vi "sid_output.vi"(6 "inputValid":bool, 7 "startId":bool, 9 "sysIdParams":T1={"sysIdOutputRate"=100, "sysIdWaveSize"=4092, "sysIdRepetitions"=50} {"sysIdOutputRate" min=10}, 11 "feedbackHeight":fxp<+/-,28,1>) -> (0 "sysIdRunning":bool, 1 "recordPoint":bool, 2 "sysIdRep":u16, 3 "sid.o.height":fxp<+/-,28,1>, 4 "outputValid":bool)   [LabVIEW 2016]
uses:
  <vilib>/rvi/DataTransferAndStorage/Container/XNode/niFpgaContainer.xnode
  <instrlib>/_niInstr/Basic Elements/v1/FPGA/niInstr Basic Elements v1 FPGA.lvlib
  <vilib>/rvi/FXPMathLib/FxpAdd/XNode/nifxpmath_Add.xnode
  <vilib>/rvi/FXPMathLib/sim/FxpSim.dll
  <vilib>/rvi/FXPMathLib/FxpInterpret/XNode/nifxpmath_Interpret.xnode
  <vilib>/rvi/Memory/Memory_Emulation/nirvimemoryFastEmulation.vi
  <vilib>/rvi/Memory/Memory_Emulation/nirvimemoryEmulation.vi
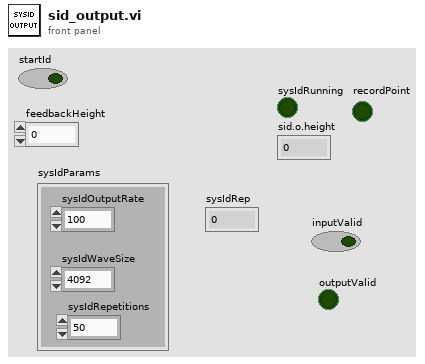
[diagram p1: front panel]
types:
  T1 = cluster{"sysIdOutputRate":u16, "sysIdWaveSize":u16, "sysIdRepetitions":u16}
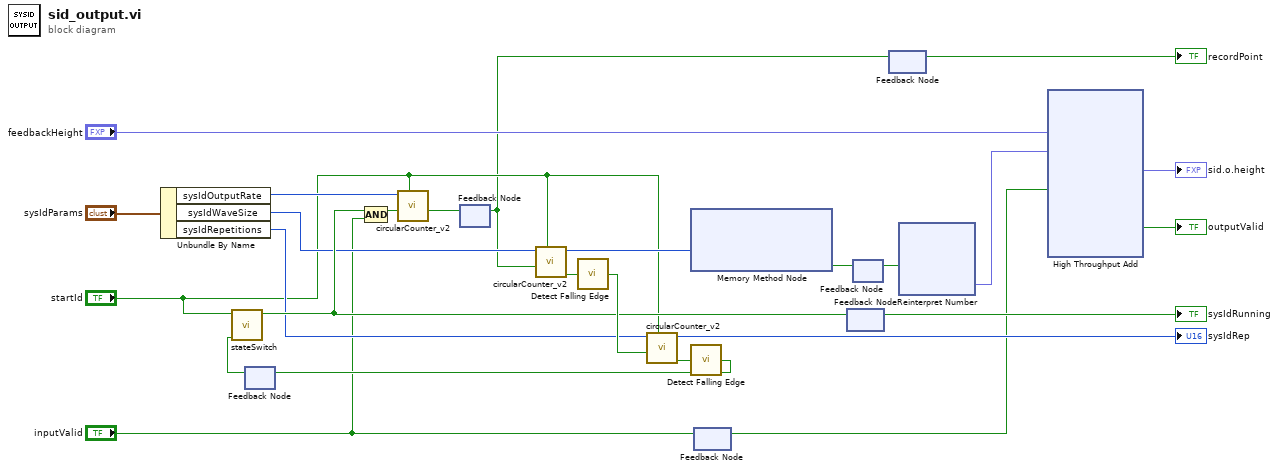
[diagram p0: block diagram]
diagram:
  n1 = Unbundle By Name("sysIdParams") -> ("sysIdOutputRate"=w17:u16, "sysIdWaveSize"=w16:u16, "sysIdRepetitions"=w15:u16)
  n2 = feedback #1() -> (w21:bool)  [unwired: 1 in]
  n3 = call "stateSwitch.vi"("disable"=w21, "enable"="startId") -> ("state"=w19:bool)  [unwired: 9 in]
  n4 = Compound Arithmetic op=AND(w19, "inputValid") -> (w5:bool)
  n5 = call "circularCounter_v2.vi"("reset"="startId", "doStep"=w5, "maxCount"=w17) -> ("maxPulse"=w6:bool)  [unwired: 5 in, 3 out]
  n6 = feedback-in #2(w6) -> ()
  n7 = feedback #2() -> (w4:bool)  [unwired: 1 in]
  n8 = call "circularCounter_v2.vi"("reset"="startId", "doStep"=w4, "maxCount"=w16) -> ("maxReached"=w25:bool, "index"=w26:u16)  [unwired: 5 in, 2 out]
  n9 = call <instrlib>:"Detect Falling Edge.vi"("signal"=w25) -> ("edge detected"=w24:bool)  [unwired: 14 in]
  n10 = call "circularCounter_v2.vi"("reset"="startId", "doStep"=w24, "maxCount"=w15) -> ("maxReached"=w23:bool, "index"=→"sysIdRep":u16)  [unwired: 5 in, 2 out]
  n11 = xnode ("Memory Method Node")("Address"=w26) -> ("Data"=w20:bool)  [unwired: 1 in, 1 out]
  n12 = call <instrlib>:"Detect Falling Edge.vi"("signal"=w23) -> ("edge detected"=w22:bool)  [unwired: 14 in]
  n13 = feedback-in #1(w22) -> ()
  n14 = feedback #3() -> (w2:bool)  [unwired: 1 in]
  n15 = feedback-in #3("inputValid") -> ()
  n16 = feedback #4() -> (→"sysIdRunning":bool)  [unwired: 1 in]
  n17 = feedback-in #4(w19) -> ()
  n18 = feedback #5() -> (w9:bool)  [unwired: 1 in]
  n19 = feedback-in #5(w20) -> ()
  n20 = feedback-in #6(w4) -> ()
  n21 = feedback #6() -> (→"recordPoint":bool)  [unwired: 1 in]
  n22 = xnode "Reinterpret Number"("x"=w9) -> ("y"=w8:fxp<+/-,16,1>)
  n23 = xnode ("High Throughput Add")("x"="feedbackHeight", "y"=w8, "input valid"=w2) -> ("x+y"=→"sid.o.height":fxp<+/-,28,1>, "output valid"=→"outputValid":bool)  [unwired: 1 in, 1 out]
